vi "Init.vi"(10 "Game Board Components[2] in":refnum<class "Game Board Component.lvclass">[](array[class]), 11 "Collision in":refnum<class "Collision.lvclass">) -> (3 "Collision out":refnum<class "Collision.lvclass">)   [LabVIEW 2021, in "Collision.lvclass"]
doc: "MIT Licence\nCopyright (c) 2024 David Grollier"
uses:
  Collision.lvclass
  Game Componants/Game Board Component/Game Board Component.lvclass
  Collision.lvclass/Collision.ctl
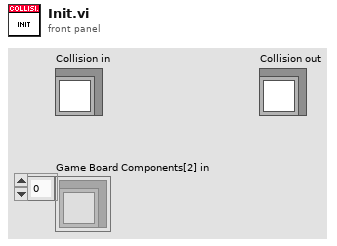
[diagram p1: front panel]
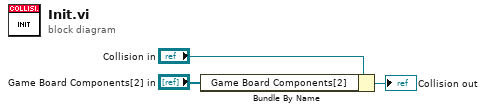
[diagram p0: block diagram]
diagram:
  n1 = Bundle By Name(cluster="Collision in", "Game Board Components[2]"="Game Board Components[2] in") -> (→"Collision out":refnum<class "Collision.lvclass">)
